vi "GetAttributeViReal64_SA-Gating_Sweep.vi"(8 "error in (no error)":errorcluster {"code" format="%.0x"}, 9 "AttributeID":u32(ring)=1150526 items=["SA_GATING_DELAY"=1150526, "SA_GATING_HOLD_OFF_TIME"=1150535, "SA_GATING_LENGTH"=1150528, "SA_GATING_MIN_FAST"=1150530, "SA_GATING_VIEW_START_TIME"=1150875, "SA_GATING_VIEW_SWEEP_TIME"=1150534, "SA_SWEEPCOUPLING_BANDWIDTH_RATIO"=1150722, "SA_SWEEPCOUPLING_FFT_WIDTH"=1150725, "SA_SWEEPCOUPLING_FFT_WIDTH_TO_SPAN_RATIO"=1150727], 11 "instrument handle":refnum<k15>) -> (0 "error out":errorcluster {"code" format="%.0x"}, 2 "AttributeValue":dbl, 3 "instrument handle out":refnum<k15>)   [LabVIEW 2009, in "Keysight XSAn.lvlib"]
doc: "Gets a Real64 attribute from the instrument driver.\nThe following Attributes are supported:\n\nSA_GATING_DELAY\nSA_GATING_HOLD_OFF_TIME\nSA_GATING_LENGTH\nSA_GATING_MIN_FAST\nSA_GATING_VIEW_START_TIME\nSA_GATING_VIEW_SWEEP_TIME\nSA_SWEEPCOUPLING_BANDWIDTH_RATIO\nSA_SWEEPCOUPLING_FFT_WIDTH\nSA_SWEEPCOUPLING_FFT_WIDTH_TO_SPAN_RATIO"
uses:
  <instrlib>/Keysight XSAn/Keysight XSAn.lvlib
  AgXSAn.dll
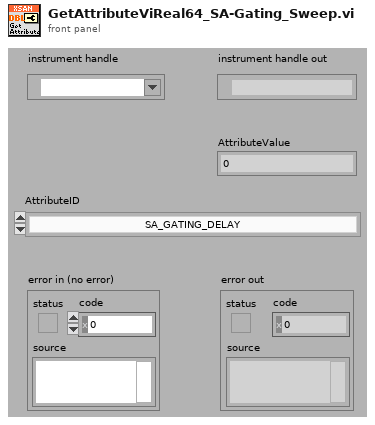
[diagram p1: front panel]
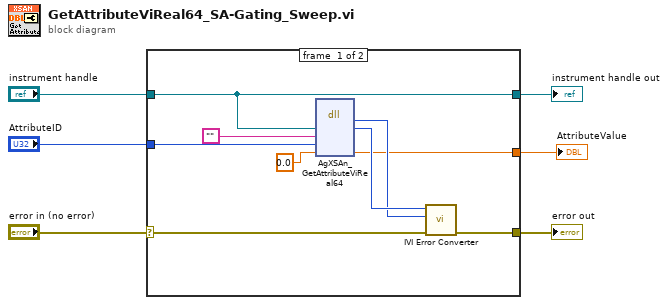
[diagram p0: block diagram]
diagram:
  n1 = case shown="No Error" "error in (no error)" {
    selector: "error in (no error)" -> [w13 w17]
    tunnel: [w12 w17] -> w6
    tunnel: "instrument handle" -> [w8 w16]
    tunnel: "AttributeID" -> [w11 _]
    tunnel: [w9 _] -> w2
    tunnel: [w8 w16] -> w1
    frame #0 {
      n2 = dll-call lib="AgXSAn**.dll" fn="AgXSAn_GetAttributeViReal64"("Vi"=w8, "RepCapIdentifier"="", "AttributeID"=w11, "AttributeValue"=0.0) -> ("return type"=w14:i32, "Vi"=w15:u32, "AttributeValue"=w9:dbl)  [unwired: 5 in, 2 out]
      n3 = call <instrlib>:"IVI Error Converter.vi"("error in (no error)"=w13, "IVI error code (0)"=w14, "instrument handle"=w15) -> ("error out"=w12:errorcluster)  [unwired: 7 in, 1 out]
    }
    frame #1 {
    }
  }
  "error out" <- w6
  "instrument handle out" <- w1
  "AttributeValue" <- w2
